vi "PickNDrop.vi"(6 "Options":T1(ring)=enum."DropTool", 9 "Z":dbl format="%#_13g", 10 "Y":dbl=977.82 format="%#_13g", 11 "X":dbl=276.904 format="%#_13g") -> (0 "error out":errorcluster, 5 "controller out":refnum<k24>)   [LabVIEW 2016]
uses:
  C:/Users/TTUHEP/Documents/LabVIEW/Other Models/2010/Bin/Aerotech.A3200.dll
  Other Models/2010/Bin/Aerotech.A3200.dll
  Other Models/2010/Motion/AbortSingle.vi
panel:
  out "element":bool
  out "Numeric":i32
  out "Boolean":bool
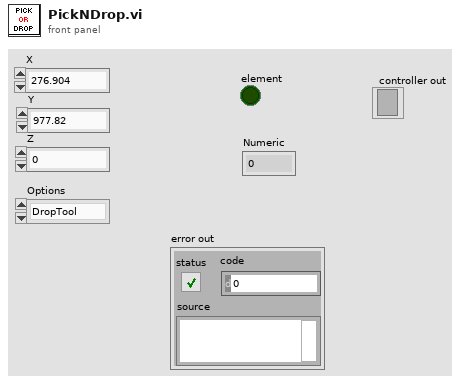
[diagram p1: front panel]
types:
  T1 = enum16{"PickTool", "DropTool", "PickPlate", "DropPlate"}
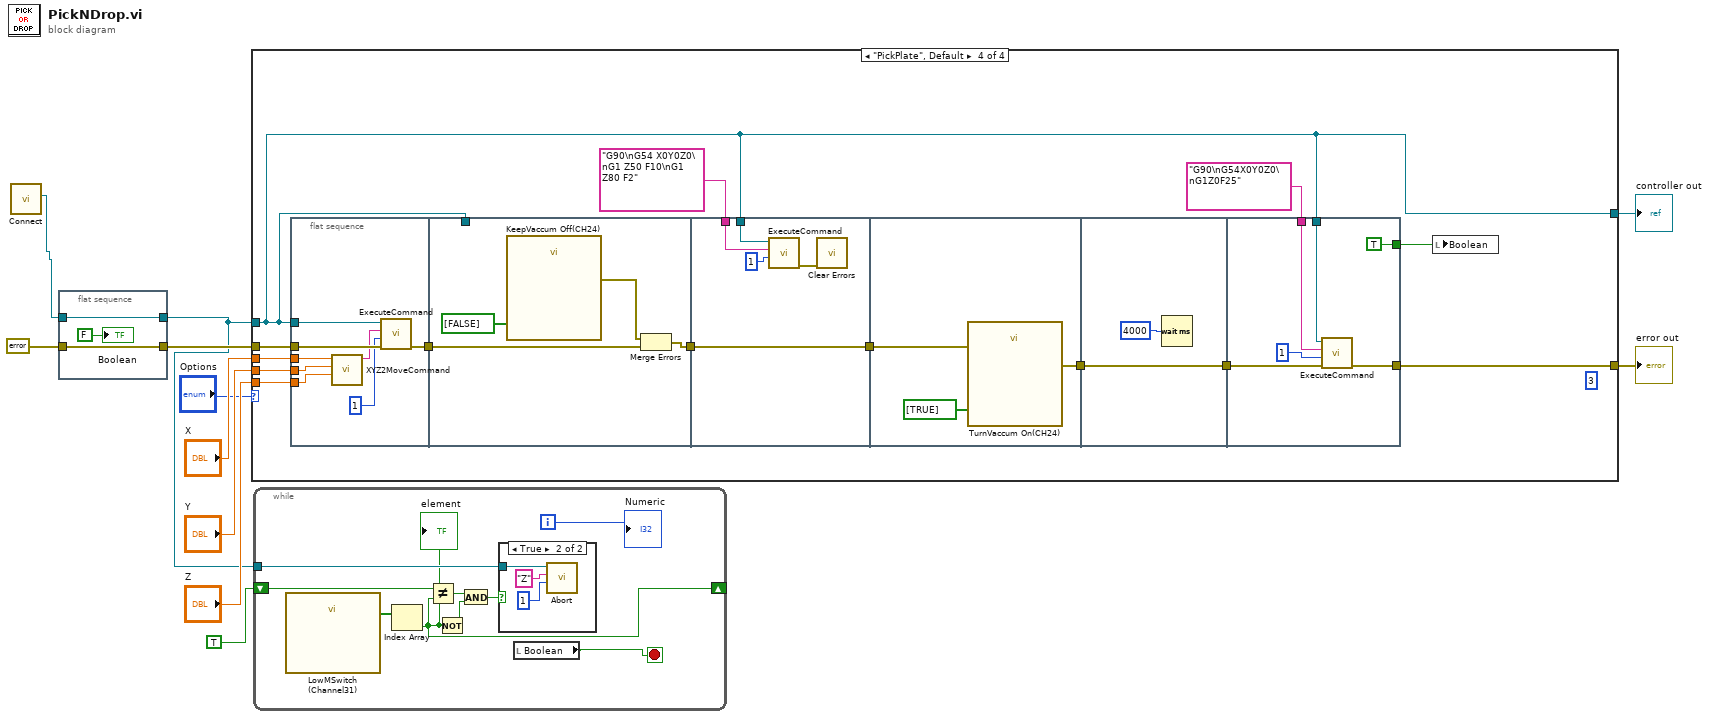
[diagram p0: block diagram]
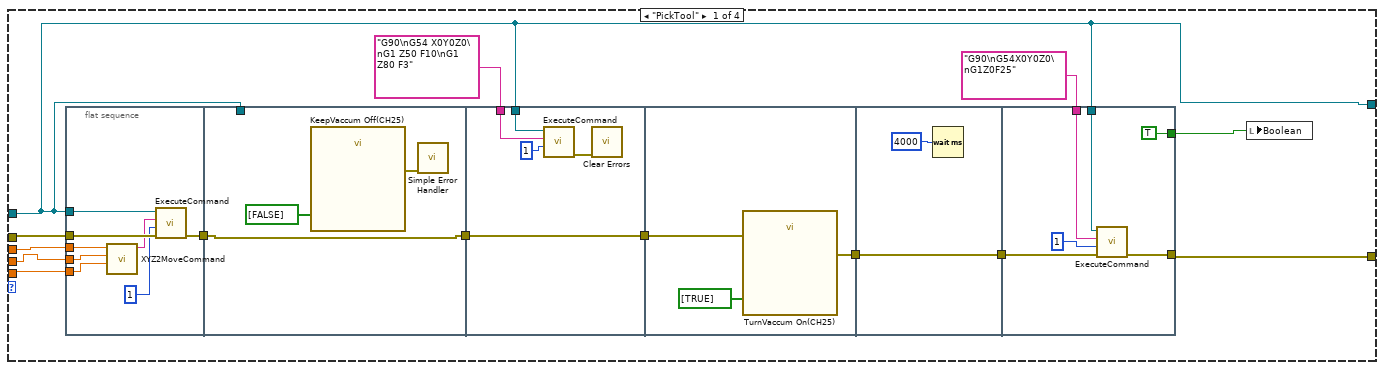
[diagram p3: hidden frame]
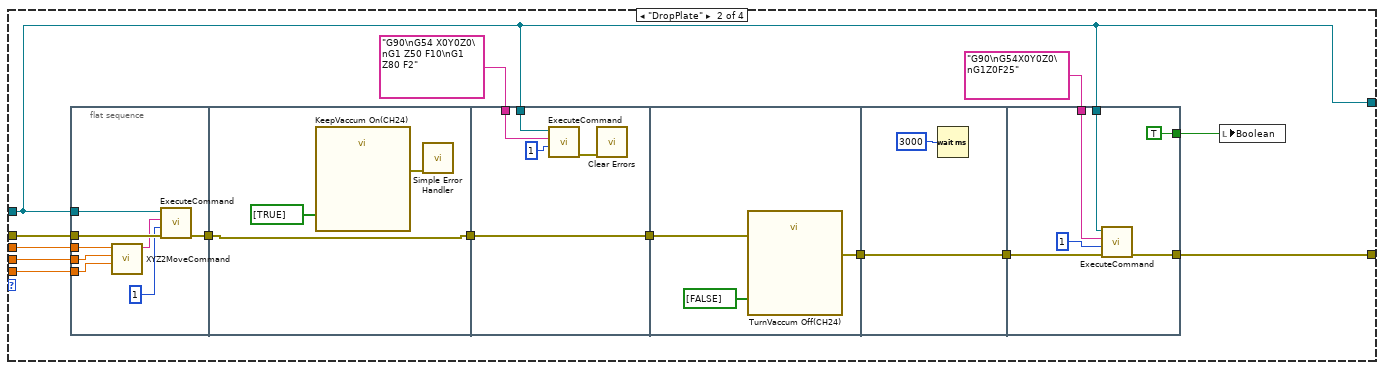
[diagram p4: hidden frame]
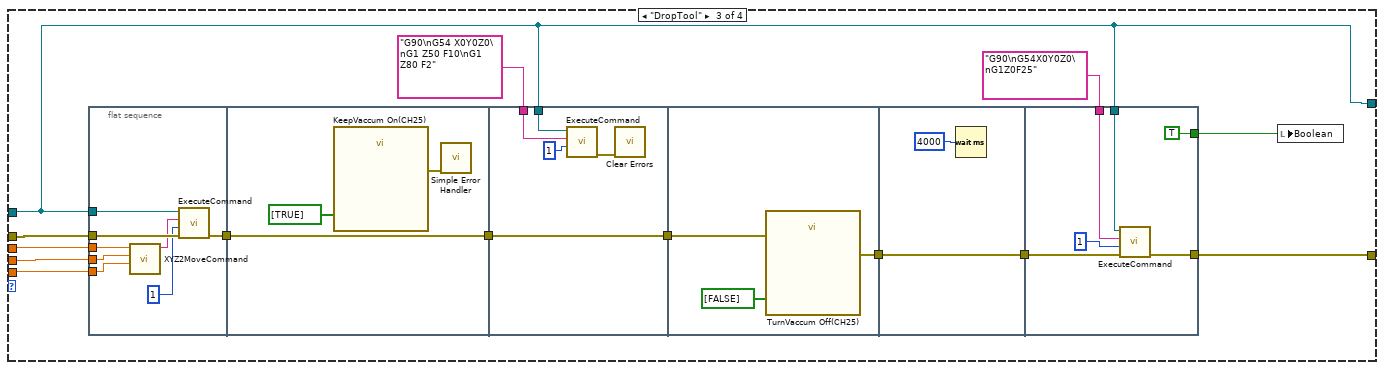
[diagram p5: hidden frame]
diagram:
  n1 = call "Connect.vi"() -> ("controller"=w2:refnum<k24>)  [unwired: 10 in, 1 out]
  n2 = flat-sequence {
    tunnel: errorcluster {"status"=FALSE, "code"=0, "source"=""} ("error out") -> [w14]
    tunnel: [w14] -> w6
    tunnel: w2 -> [w12]
    tunnel: [w12] -> w3
    frame #0 {
      "Boolean" <- FALSE
    }
  }
  n3 = case shown="\"PickPlate\", Default" "Options" {
    tunnel: "Z" -> [w18 w61 w100 w146]
    tunnel: "Y" -> [w19 w60 w101 w147]
    tunnel: "X" -> [w20 w59 w102 w145]
    tunnel: w6 -> [w21 w58 w103 w151]
    tunnel: w3 -> [w17 w56 w99 w139]
    tunnel: [w16 w62 w98 w148] -> w7
    tunnel: [w17 w56 w99 w139] -> w8
    frame "PickTool" {
      n4 = flat-sequence {
        tunnel: w21 -> [w36]
        tunnel: w20 -> [w33]
        tunnel: w19 -> [w32]
        tunnel: w18 -> [w31]
        tunnel: w17 -> [w30]
        tunnel: [w34] -> w28
        tunnel: [w37] -> w27
        tunnel: w17 -> [_]
        tunnel: w28 -> [w37]
        tunnel: w27 -> [w41]
        tunnel: [w41] -> w26
        tunnel: "G90\nG54 X0Y0Z0\nG1 Z50 F10\nG1 Z80 F3" -> [w44]
        tunnel: w17 -> [w43]
        tunnel: w26 -> [w47]
        tunnel: [w46] -> w25
        tunnel: w25 -> [w49]
        tunnel: [w49] -> w24
        tunnel: w17 -> [w55]
        tunnel: w24 -> [w54]
        tunnel: [w53] -> w16
        tunnel: "G90\nG54X0Y0Z0\nG1Z0F25" -> [w51]
        tunnel: [TRUE] -> w15
        frame #0 {
          n5 = call "XYZ2MoveCommand.vi"("Z"=w31, "Y"=w32, "X"=w33) -> ("String"=w29:string)  [unwired: 8 in]
          n6 = call "ExecuteCommand.vi"("error in (no error)"=w36, "taskId"=1, "Command Code"=w29, "controller in"=w30) -> ("error out"=w34:errorcluster)  [unwired: 5 in, 2 out]
        }
        frame #1 {
          n7 = call "KeepVaccum Off(CH25)"("data"=bool[] [FALSE]) -> ("error out"=w38:errorcluster)  [unwired: 17 in, 1 out]
          n8 = call <vilib>:"Simple Error Handler.vi"("error in (no error)"=w38) -> ()  [unwired: 4 in, 5 out]
        }
        frame #2 {
          n9 = call "ExecuteCommand.vi"("taskId"=1, "Command Code"=w44, "controller in"=w43) -> ("error out"=w40:errorcluster)  [unwired: 6 in, 2 out]
          n10 = call <vilib>:"Clear Errors.vi"("error in (no error)"=w40) -> ()  [unwired: 5 in, 2 out]
        }
        frame #3 {
          n11 = call "TurnVaccum On(CH25)"("data"=bool[] [TRUE], "error in"=w47) -> ("error out"=w46:errorcluster)  [unwired: 16 in, 1 out]
        }
        frame #4 {
          n12 = Wait (ms)(milliseconds to wait=4000) -> ()  [unwired: 1 out]
        }
        frame #5 {
          n13 = call "ExecuteCommand.vi"("error in (no error)"=w54, "taskId"=1, "Command Code"=w51, "controller in"=w55) -> ("error out"=w53:errorcluster)  [unwired: 5 in, 2 out]
        }
      }
      n14 = local write "Boolean"(w15) -> ()
    }
    frame "DropPlate" {
      n15 = flat-sequence {
        tunnel: w58 -> [w77]
        tunnel: w59 -> [w74]
        tunnel: w60 -> [w73]
        tunnel: w61 -> [w72]
        tunnel: w56 -> [w71]
        tunnel: [w75] -> w69
        tunnel: [w78] -> w68
        tunnel: w69 -> [w78]
        tunnel: w68 -> [w82]
        tunnel: [w82] -> w67
        tunnel: "G90\nG54 X0Y0Z0\nG1 Z50 F10\nG1 Z80 F2" -> [w85]
        tunnel: w56 -> [w84]
        tunnel: w67 -> [w88]
        tunnel: [w87] -> w66
        tunnel: w66 -> [w90]
        tunnel: [w90] -> w65
        tunnel: w56 -> [w96]
        tunnel: w65 -> [w95]
        tunnel: [w94] -> w62
        tunnel: "G90\nG54X0Y0Z0\nG1Z0F25" -> [w92]
        tunnel: [TRUE] -> w57
        frame #0 {
          n16 = call "XYZ2MoveCommand.vi"("Z"=w72, "Y"=w73, "X"=w74) -> ("String"=w70:string)  [unwired: 8 in]
          n17 = call "ExecuteCommand.vi"("error in (no error)"=w77, "taskId"=1, "Command Code"=w70, "controller in"=w71) -> ("error out"=w75:errorcluster)  [unwired: 5 in, 2 out]
        }
        frame #1 {
          n18 = call "KeepVaccum On(CH24)"("data"=bool[] [TRUE]) -> ("error out"=w79:errorcluster)  [unwired: 17 in, 1 out]
          n19 = call <vilib>:"Simple Error Handler.vi"("error in (no error)"=w79) -> ()  [unwired: 4 in, 5 out]
        }
        frame #2 {
          n20 = call "ExecuteCommand.vi"("taskId"=1, "Command Code"=w85, "controller in"=w84) -> ("error out"=w81:errorcluster)  [unwired: 6 in, 2 out]
          n21 = call <vilib>:"Clear Errors.vi"("error in (no error)"=w81) -> ()  [unwired: 5 in, 2 out]
        }
        frame #3 {
          n22 = call "TurnVaccum Off(CH24)"("data"=bool[] [FALSE], "error in"=w88) -> ("error out"=w87:errorcluster)  [unwired: 16 in, 1 out]
        }
        frame #4 {
          n23 = Wait (ms)(milliseconds to wait=3000) -> ()  [unwired: 1 out]
        }
        frame #5 {
          n24 = call "ExecuteCommand.vi"("error in (no error)"=w95, "taskId"=1, "Command Code"=w92, "controller in"=w96) -> ("error out"=w94:errorcluster)  [unwired: 5 in, 2 out]
        }
      }
      n25 = local write "Boolean"(w57) -> ()
    }
    frame "DropTool" {
      n26 = flat-sequence {
        tunnel: w103 -> [w118]
        tunnel: w102 -> [w115]
        tunnel: w101 -> [w114]
        tunnel: w100 -> [w113]
        tunnel: w99 -> [w112]
        tunnel: [w116] -> w110
        tunnel: [w119] -> w109
        tunnel: w110 -> [w119]
        tunnel: w109 -> [w123]
        tunnel: [w123] -> w108
        tunnel: "G90\nG54 X0Y0Z0\nG1 Z50 F10\nG1 Z80 F2" -> [w126]
        tunnel: w99 -> [w125]
        tunnel: w108 -> [w129]
        tunnel: [w128] -> w107
        tunnel: w107 -> [w131]
        tunnel: [w131] -> w106
        tunnel: w99 -> [w137]
        tunnel: w106 -> [w136]
        tunnel: [w135] -> w98
        tunnel: "G90\nG54X0Y0Z0\nG1Z0F25" -> [w133]
        tunnel: [TRUE] -> w97
        frame #0 {
          n27 = call "XYZ2MoveCommand.vi"("Z"=w113, "Y"=w114, "X"=w115) -> ("String"=w111:string)  [unwired: 8 in]
          n28 = call "ExecuteCommand.vi"("error in (no error)"=w118, "taskId"=1, "Command Code"=w111, "controller in"=w112) -> ("error out"=w116:errorcluster)  [unwired: 5 in, 2 out]
        }
        frame #1 {
          n29 = call "KeepVaccum On(CH25)"("data"=bool[] [TRUE]) -> ("error out"=w120:errorcluster)  [unwired: 17 in, 1 out]
          n30 = call <vilib>:"Simple Error Handler.vi"("error in (no error)"=w120) -> ()  [unwired: 4 in, 5 out]
        }
        frame #2 {
          n31 = call "ExecuteCommand.vi"("taskId"=1, "Command Code"=w126, "controller in"=w125) -> ("error out"=w122:errorcluster)  [unwired: 6 in, 2 out]
          n32 = call <vilib>:"Clear Errors.vi"("error in (no error)"=w122) -> ()  [unwired: 5 in, 2 out]
        }
        frame #3 {
          n33 = call "TurnVaccum Off(CH25)"("data"=bool[] [FALSE], "error in"=w129) -> ("error out"=w128:errorcluster)  [unwired: 16 in, 1 out]
        }
        frame #4 {
          n34 = Wait (ms)(milliseconds to wait=4000) -> ()  [unwired: 1 out]
        }
        frame #5 {
          n35 = call "ExecuteCommand.vi"("error in (no error)"=w136, "taskId"=1, "Command Code"=w133, "controller in"=w137) -> ("error out"=w135:errorcluster)  [unwired: 5 in, 2 out]
        }
      }
      n36 = local write "Boolean"(w97) -> ()
    }
    frame "PickPlate", Default {
      (unwired) 3
      n37 = flat-sequence {
        tunnel: w151 -> [w159]
        tunnel: w145 -> [w156]
        tunnel: w147 -> [w155]
        tunnel: w146 -> [w154]
        tunnel: w139 -> [w152]
        tunnel: [w157] -> w150
        tunnel: [w160] -> w149
        tunnel: w139 -> [_]
        tunnel: w150 -> [w162]
        tunnel: w149 -> [w165]
        tunnel: [w165] -> w144
        tunnel: "G90\nG54 X0Y0Z0\nG1 Z50 F10\nG1 Z80 F2" -> [w168]
        tunnel: w139 -> [w167]
        tunnel: w144 -> [w171]
        tunnel: [w170] -> w143
        tunnel: w143 -> [w173]
        tunnel: [w173] -> w142
        tunnel: w139 -> [w179]
        tunnel: w142 -> [w178]
        tunnel: [w177] -> w148
        tunnel: "G90\nG54X0Y0Z0\nG1Z0F25" -> [w175]
        tunnel: [TRUE] -> w138
        frame #0 {
          n38 = call "XYZ2MoveCommand.vi"("Z"=w154, "Y"=w155, "X"=w156) -> ("String"=w153:string)  [unwired: 8 in]
          n39 = call "ExecuteCommand.vi"("error in (no error)"=w159, "taskId"=1, "Command Code"=w153, "controller in"=w152) -> ("error out"=w157:errorcluster)  [unwired: 5 in, 2 out]
        }
        frame #1 {
          n40 = call "KeepVaccum Off(CH24)"("data"=bool[] [FALSE]) -> ("error out"=w161:errorcluster)  [unwired: 17 in, 1 out]
          n41 = Merge Errors(w161, w162) -> (w160:errorcluster)
        }
        frame #2 {
          n42 = call "ExecuteCommand.vi"("taskId"=1, "Command Code"=w168, "controller in"=w167) -> ("error out"=w164:errorcluster)  [unwired: 6 in, 2 out]
          n43 = call <vilib>:"Clear Errors.vi"("error in (no error)"=w164) -> ()  [unwired: 5 in, 2 out]
        }
        frame #3 {
          n44 = call "TurnVaccum On(CH24)"("data"=bool[] [TRUE], "error in"=w171) -> ("error out"=w170:errorcluster)  [unwired: 16 in, 1 out]
        }
        frame #4 {
          n45 = Wait (ms)(milliseconds to wait=4000) -> ()  [unwired: 1 out]
        }
        frame #5 {
          n46 = call "ExecuteCommand.vi"("error in (no error)"=w178, "taskId"=1, "Command Code"=w175, "controller in"=w179) -> ("error out"=w177:errorcluster)  [unwired: 5 in, 2 out]
        }
      }
      n47 = local write "Boolean"(w138) -> ()
    }
  }
  "controller out" <- w8
  "error out" <- w7
  n48 = while {
    tunnel: w3 -> [w188]
    shift-right: [w183] -> _
    shift-left: TRUE -> [w186]
    i -> [w180]
    stop <- w181 stop-if-true
    n49 = call "LowMSwitch     (Channel31)"() -> ("data"=w187:bool[])  [unwired: 17 in, 2 out]
    n50 = Index Array(array=w187) -> (element=w183:bool)  [unwired: 1 in]
    "element" <- w183
    n51 = Not Equal?(x=w186, y=w183) -> (x != y?=w184:bool)
    n52 = Not(x=w183) -> (.not. x?=w182:bool)
    n53 = And(x=w184, y=w182) -> (x .and. y?=w185:bool)
    n54 = case shown="True" w185 {
      tunnel: w188 -> [_ w191]
      frame False {
      }
      frame True {
        n55 = call-poly "Abort.vi"("taskId"=1, "axis name? (all)"="Z", "controller in"=w191) -> ()  [unwired: 7 in, 2 out]
      }
    }
    n56 = local read "Boolean"() -> (w181:bool)
    "Numeric" <- w180
  }
